vi "HKey Classes Root Key Read DWord.vi"(4 "error in (no error)":errorcluster, 5 "registry view":T1 items=["Default"=0, "KEY_WOW64_64KEY"=8, "KEY_WOW64_32KEY"=9], 6 "registry search value":string, 7 "registry search key":string) -> (0 "error out":errorcluster, 2 "result data type":T2(ring), 3 "result of registry search":u32)   [LabVIEW 2017]
doc: "Read access to a DIAdem registry entry."
uses:
  <vilib>/registry/registry.llb/Registry View.ctl
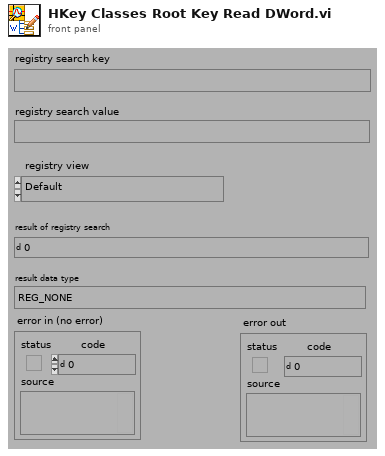
[diagram p1: front panel]
types:
  T1 = typedef "Registry View.ctl" = u16
  T2 = enum32{"REG_NONE", "REG_SZ", "REG_EXPAND_SZ", "REG_BINARY", "REG_DWORD_LITTLE_ENDIAN", "REG_DWORD_BIG_ENDIAN", "REG_LINK", "REG_MULTI_SZ", "REG_RESOURCE_LIST", "REG_FULL_RESOURCE_DESCRIPTOR", "REG_RESOURCE_REQUIREMENTS_LIST"}
  T3 = enum16{"KEY_QUERY_VALUE", "KEY_SET_VALUE", "KEY_CREATE_SUB_KEY", "KEY_ENUMERATE_SUB_KEYS", "KEY_NOTIFY", "KEY_CREATE_LINK", "KEY_READ", "KEY_WRITE", "KEY_ALL_ACCESS"}
  T4 = enum16{"HKEY_CLASSES_ROOT", "HKEY_CURRENT_USER", "HKEY_LOCAL_MACHINE", "HKEY_USERS", "HKEY_PERFORMANCE_DATA", "HKEY_CURRENT_CONFIG", "HKEY_DYN_DATA"}
  T5 = typedef "Registry refnum.ctl" = refnum<k1>
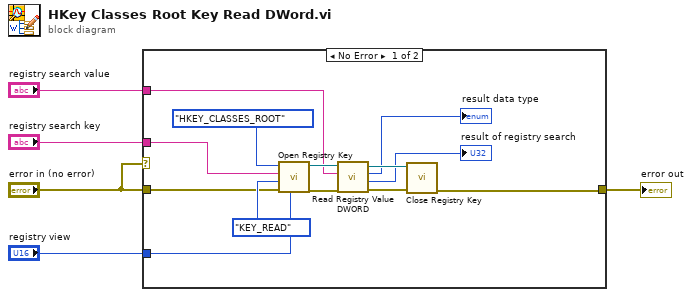
[diagram p0: block diagram]
diagram:
  n1 = case shown="No Error" "error in (no error)" {
    tunnel: "registry search key" -> [w9 _]
    tunnel: [w7 w19] -> w4
    tunnel: "error in (no error)" -> [w8 w19]
    tunnel: "registry search value" -> [w10 _]
    tunnel: "registry view" -> [w6 _]
    frame No Error {
      n2 = call <vilib>:"Open Registry Key.vi"("registry view"=w6, "error in (no error)"=w8, "security access mask (KEY_READ | KEY_WRITE)"=T3."KEY_READ" ("security access mask (all)"), "subkey"=w9, "root key (HKEY_LOCAL_MACHINE)"=T4."HKEY_CLASSES_ROOT" ("root key")) -> ("error out"=w15:errorcluster, "refnum out"=w16:T5)  [unwired: 5 in]
      n3 = call <vilib>:"Read Registry Value DWORD.vi"("error in (no error)"=w15, "value"=w10, "refnum"=w16) -> ("error out"=w13:errorcluster, "DWORD data"=→"result of registry search":u32, "data type"=→"result data type":T2, "refnum out"=w14:T5)  [unwired: 5 in]
      n4 = call <vilib>:"Close Registry Key.vi"("error in (no error)"=w13, "refnum"=w14) -> ("error out"=w7:errorcluster)  [unwired: 5 in]
    }
    frame Error {
    }
  }
  "error out" <- w4
